vi "Launch.vi"(8 "error in":errorcluster, 11 "Philips Subpanel in":refnum<class "Flex UI Subpanel.lvclass">) -> (0 "error out":errorcluster, 3 "Philips Subpanel out":refnum<class "Flex UI Subpanel.lvclass">)   [LabVIEW 2014, in "Flex UI Subpanel.lvclass"]
doc: "Launches the UI."
uses:
  Flex UI Subpanel.lvclass
  Flex UI (Parent)/Flex UI.lvclass
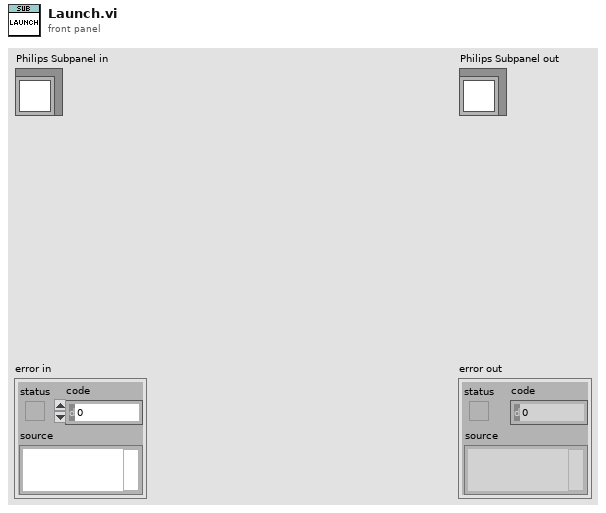
[diagram p1: front panel]
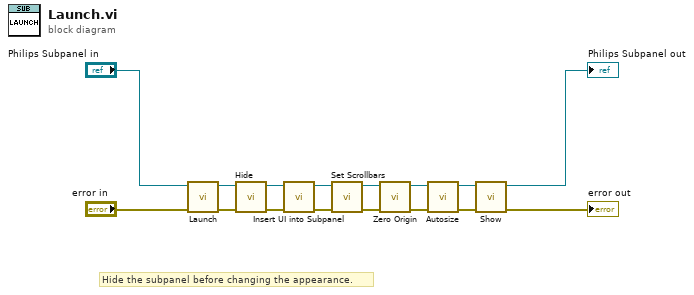
[diagram p0: block diagram]
diagram:
  # "Hide the subpanel before changing the appearance."
  n1 = call-parent "Launch.vi"("error in"="error in", "Philips UI in"="Philips Subpanel in") -> ("error out"=w3:errorcluster, "Philips UI out"=w1:refnum<class "Flex UI Subpanel.lvclass">)  [unwired: 8 in]
  n2 = call-dynamic "Hide.vi"("error in"=w3, "Philips Subpanel in"=w1) -> ("error out"=w16:errorcluster, "Philips Subpanel out"=w10:refnum<class "Flex UI Subpanel.lvclass">)  [unwired: 8 in]
  n3 = call "Insert UI into Subpanel.vi"("error in"=w16, "Philips Subpanel in"=w10) -> ("error out"=w14:errorcluster, "Philips Subpanel out"=w12:refnum<class "Flex UI Subpanel.lvclass">)  [unwired: 8 in]
  n4 = call "Set Scrollbars.vi"("error in"=w14, "Philips Subpanel in"=w12) -> ("error out"=w13:errorcluster, "Philips Subpanel out"=w11:refnum<class "Flex UI Subpanel.lvclass">)  [unwired: 8 in]
  n5 = call "Zero Origin.vi"("error in"=w13, "Philips UI in"=w11) -> ("error out"=w7:errorcluster, "Philips UI out"=w5:refnum<class "Flex UI Subpanel.lvclass">)  [unwired: 8 in]
  n6 = call "Autosize.vi"("error in"=w7, "Philips Subpanel in"=w5) -> ("error out"=w6:errorcluster, "Philips Subpanel out"=w4:refnum<class "Flex UI Subpanel.lvclass">)  [unwired: 8 in]
  n7 = call-dynamic "Show.vi"("error in"=w6, "Philips Subpanel in"=w4) -> ("error out"=→"error out":errorcluster, "Philips Subpanel out"=→"Philips Subpanel out":refnum<class "Flex UI Subpanel.lvclass">)  [unwired: 8 in]
